vi "pf_Set_Acquisition_Window.vi"(8 "error in (no error)":errorcluster, 11 "IMAQ Session in":refnum<k11>) -> (0 "error out":errorcluster, 2 "Data Resolution":string, 3 "IMAQ Session out":refnum<k11>)   [LabVIEW 2025, in "Photonfocus_Toolkit.lvlib"]
doc: "Sets the NI framegrabber acquisition window based on camera acquisition settings."
uses:
  Photonfocus_Toolkit.lvlib
  _Private/Controls/pf_Camera_ctrl_mngr_action.ctl
  _Private/Controls/pf_PeakDetector_Mode.ctl
  _Public/SubVIs/pf_Get_Camera_Property_Mode.vi
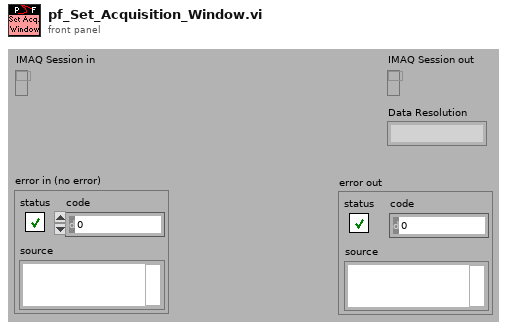
[diagram p1: front panel]
types:
  T1 = typedef "Photonfocus_Toolkit.lvlib/pf_Camera_ctrl_mngr_action.ctl" = enum16{"Create", "Destroy", "Set", "Get"}
  T2 = typedef "Photonfocus_Toolkit.lvlib/pf_PeakDetector_Mode.ctl" = enum16{"Undefined", "2D only", "2D and 3D", "3D only"}
  T3 = typedef "Photonfocus_Toolkit.lvlib/pf_Camera_Control.ctl" = cluster{"Port Name":string, "Port Number":i32, "IMAQ Session":refnum<k11>, "PeakDetector_Mode":T2, "Window.W":u32, "Window.H":u32}
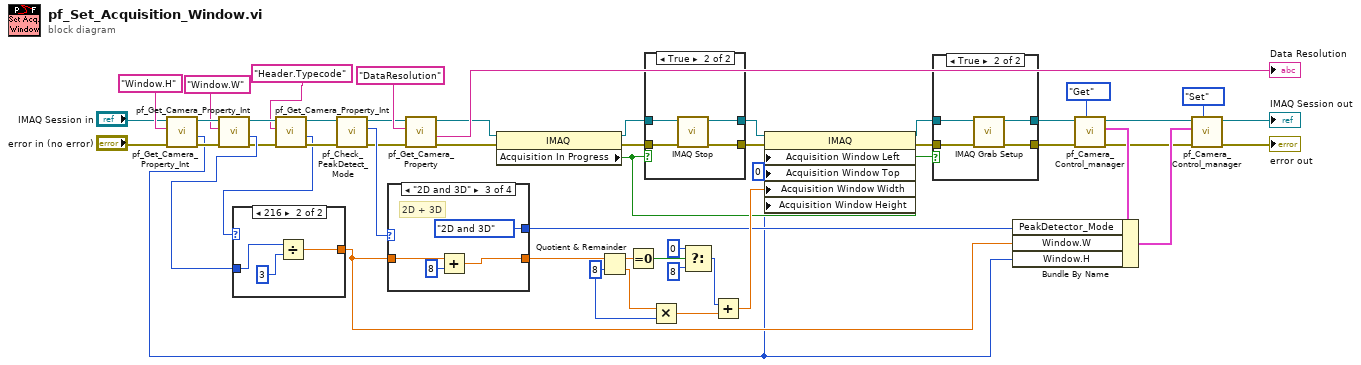
[diagram p0: block diagram]
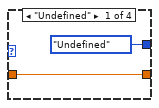
[diagram p5: hidden frame]
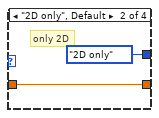
[diagram p6: hidden frame]
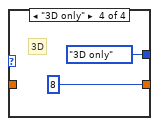
[diagram p7: hidden frame]
diagram:
  w41 = u32 0 ("Acquisition Parameters : Acquisition Window : Left")
  w50 = u32 8 ("y")
  n1 = call "pf_Get_Camera_Property_Int.vi"("error in (no error)"="error in (no error)", "Property Name"="Window.H" ("pProperty"), "IMAQ Session in"="IMAQ Session in") -> ("error out"=w42:errorcluster, "Property Value"=w8:i32, "IMAQ Session out"=w39:refnum<k11>)  [unwired: 6 out]
  n2 = call "pf_Get_Camera_Property_Int.vi"("error in (no error)"=w42, "Property Name"="Window.W" ("pProperty"), "IMAQ Session in"=w39) -> ("error out"=w6:errorcluster, "Property Value"=w7:i32, "IMAQ Session out"=w3:refnum<k11>)  [unwired: 6 out]
  n3 = call "pf_Get_Camera_Property_Int.vi"("error in (no error)"=w6, "Property Name"="Header.Typecode" ("pProperty"), "IMAQ Session in"=w3) -> ("error out"=w5:errorcluster, "Property Value"=w2:i32, "IMAQ Session out"=w4:refnum<k11>)  [unwired: 6 out]
  n4 = case shown="216" w2 {
    tunnel: w7 -> [w52 w55]
    tunnel: [w52 w53] -> w9
    frame Default {
    }
    frame 216 {
      n5 = Divide(x=w55, y=3) -> (x/y=w53:dbl)
    }
  }
  n6 = call "pf_Check_PeakDetect_Mode.vi"("error in"=w5, "IMAQ Session in"=w4) -> ("error out"=w11:errorcluster, "PeakDetector_Mode"=w12:T2, "IMAQ Session out"=w13:refnum<k11>)  [unwired: 7 out]
  n7 = case shown="\"2D and 3D\"" w12 {
    tunnel: [w56 w59 w61 u32 8 ("Width")] -> w10
    tunnel: w9 -> [w56 w59 w62 _]
    tunnel: [pf_PeakDetector_Mode."Undefined" ("PeakDetector_Mode") pf_PeakDetector_Mode."2D only" ("PeakDetector_Mode") pf_PeakDetector_Mode."2D and 3D" ("PeakDetector_Mode") pf_PeakDetector_Mode."3D only" ("PeakDetector_Mode")] -> w22
    frame "Undefined" {
    }
    frame "2D only", Default {
      # "only 2D"
    }
    frame "2D and 3D" {
      # "2D + 3D"
      n8 = Add(x=w62, y=u32 8 ("Width")) -> (x+y=w61:dbl)
    }
    frame "3D only" {
      # "3D"
    }
  }
  n9 = call-poly "pf_Get_Camera_Property.vi"("error in (no error)"=w11, "Property Name"="DataResolution" ("pProperty"), "IMAQ Session in"=w13) -> ("error out"=w18:errorcluster, "Mode value"=→"Data Resolution":string, "IMAQ Session out"=w17:refnum<k11>)  [unwired: 6 out]
  n10 = property class="IMAQ"(reference=w17, error in=w18) -> (reference out=w16:refnum<k11>, error out=w30:errorcluster, "Acquisition In Progress"=w34:bool)
  n11 = Quotient & Remainder(x=w10, y=w50) -> (x-y*floor(x/y)=w43:dbl, floor(x/y)=w51:dbl)
  n12 = Equal To 0?(x=w43) -> (x = 0?=w44:bool)
  n13 = case shown="True" w34 {
    tunnel: w30 -> [w67 w71]
    tunnel: [w67 w70] -> w33
    tunnel: w16 -> [w66 w69]
    tunnel: [w66 w68] -> w15
    frame False {
    }
    frame True {
      n14 = call <vilib>:"IMAQ Stop.vi"("error in (no error)"=w71, "IMAQ Session In"=w69) -> ("error out"=w70:errorcluster, "IMAQ Session Out"=w68:refnum<k11>)  [unwired: 8 out]
    }
  }
  n15 = Multiply(x=w51, y=w50) -> (x*y=w49:dbl)
  n16 = Select(t=u32 0 ("y"), s=w44, f=u32 8 ("y")) -> (s? t:f=w48:u32)
  n17 = Add(x=w48, y=w49) -> (x+y=w45:dbl)
  n18 = property class="IMAQ"(reference=w15, error in=w33, "Acquisition Window Left"=w41, "Acquisition Window Top"=w41, "Acquisition Window Width"=w45, "Acquisition Window Height"=w8) -> (reference out=w31:refnum<k11>, error out=w32:errorcluster)
  n19 = case shown="True" w34 {
    tunnel: w32 -> [w73 w76]
    tunnel: [w73 w75] -> w25
    tunnel: w31 -> [w72 w77]
    tunnel: [w72 w74] -> w14
    frame False {
    }
    frame True {
      n20 = call <vilib>:"IMAQ Grab Setup.vi"("error in (no error)"=w76, "IMAQ Session In"=w77) -> ("error out"=w75:errorcluster, "IMAQ Session Out"=w74:refnum<k11>)  [unwired: 8 out]
    }
  }
  n21 = call "pf_Camera_Control_manager.vi"("Action"=pf_Camera_ctrl_mngr_action."Get", "error in (no error)"=w25, "IMAQ Session in"=w14) -> ("error out"=w19:errorcluster, "Camera Control out"=w23:T3, "IMAQ Session out"=w20:refnum<k11>)  [unwired: 1 in, 5 out]
  n22 = Bundle By Name(cluster=w23, "PeakDetector_Mode"=w22, "Window.W"=w9, "Window.H"=w8) -> (w21:T3)
  n23 = call "pf_Camera_Control_manager.vi"("Action"=pf_Camera_ctrl_mngr_action."Set", "error in (no error)"=w19, "Camera Control in"=w21, "IMAQ Session in"=w20) -> ("error out"=→"error out":errorcluster, "IMAQ Session out"=→"IMAQ Session out":refnum<k11>)  [unwired: 6 out]
